vi "Set Type Pt1000.vi"(6 "Resistance value (if 2 wires)":dbl, 8 "error in (no error)":errorcluster, 9 "Wire number":u16(ring) items=["W2", "W3"], 10 "Channel":u16(ring) items=["A1"=0, "A2"=1, "A3"=2, "A4"=3, "A5"=4, "A6"=5, "A7"=6, "A8"=7, "A9"=8, "A10"=9, "K1"=200, "K2"=201, "K3"=202, "K4"=203, "FA1"=204, "FA2"=205, "FA3"=206, "FA4"=207], 11 "VISA resource name":refnum<visa-resource-name>) -> (0 "error out":errorcluster, 3 "VISA resource name out":refnum<visa-resource-name>)   [LabVIEW 2017, in "Sefram DAS220.lvlib"]
doc: "Setup input type as Pt1000."
uses:
  <instrlib>/Sefram DAS220/Sefram DAS220.lvlib
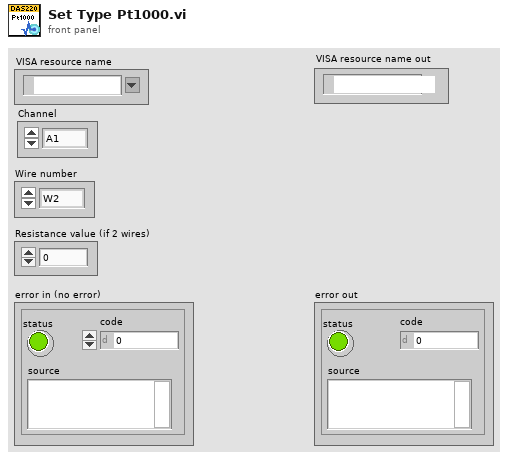
[diagram p1: front panel]
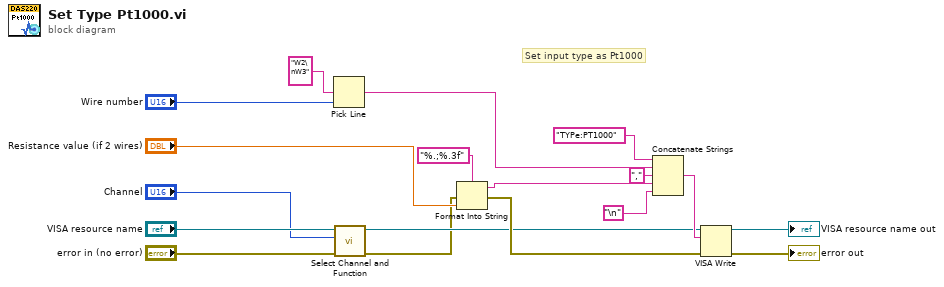
[diagram p0: block diagram]
diagram:
  # "Set input type as Pt1000"
  n1 = Pick Line(multi-line string="W2\nW3", line index="Wire number") -> (output string=w2:string)  [unwired: 1 in]
  n2 = call <instrlib>:"Select Channel and Function.vi"("error in (no error)"="error in (no error)", "Channel"="Channel", "VISA resource name"="VISA resource name") -> ("error out"=w5:errorcluster, "VISA resource name out"=w7:refnum<visa-resource-name>)  [unwired: 7 in]
  n3 = Format Into String(format string="%.;%.3f", error in=w5, "Resistance value (if 2 wires)") -> (resulting string=w12:string, error out=w11:errorcluster)  [unwired: 1 in]
  n4 = Concatenate Strings("TYPe:PT1000" ("string"), w2, "," ("string"), w12, "\n") -> (w18:string)
  n5 = VISA Write(VISA resource name=w7, write buffer=w18, error in (no error)=w11) -> (VISA resource name out=→"VISA resource name out":refnum<visa-resource-name>, error out=→"error out":errorcluster)  [unwired: 1 out]
